vi "Create Cluster Array Of Simple Arithmetic Class Instances.vi"() -> (3 "output array":T1(array[cluster]))   [LabVIEW 2012]
uses:
  ClassDefinitions/SimpleClassWithMethods/SimpleArithmetic.lvclass
panel:
  in  "Numeric":dbl=11.0
  in  "Array":T1(array[cluster])
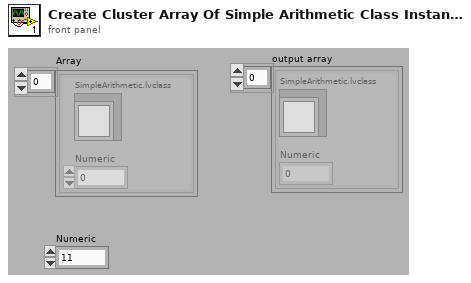
[diagram p1: front panel]
types:
  T1 = cluster{"SimpleArithmetic.lvclass":refnum<class "SimpleArithmetic.lvclass">, "Numeric":dbl}[]
  T2 = cluster{"SimpleArithmetic.lvclass":refnum<class "SimpleArithmetic.lvclass">, "Numeric":dbl}
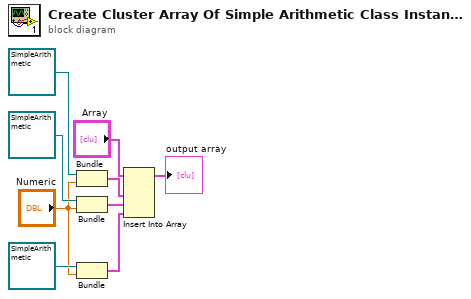
[diagram p0: block diagram]
diagram:
  n1 = Bundle("SimpleArithmetic.lvclass"=refnum<class "SimpleArithmetic.lvclass"> refnum, "Numeric"="Numeric") -> (w3:T2)  [unwired: 1 in]
  n2 = Bundle("SimpleArithmetic.lvclass"=refnum<class "SimpleArithmetic.lvclass"> refnum, "Numeric"="Numeric") -> (w2:T2)  [unwired: 1 in]
  n3 = Bundle("SimpleArithmetic.lvclass"=refnum<class "SimpleArithmetic.lvclass"> refnum, "Numeric"="Numeric") -> (w1:T2)  [unwired: 1 in]
  n4 = Insert Into Array(array="Array", new element #1=w3, new element #2=w2, new element #3=w1) -> (→"output array":T1)  [unwired: 1 in]
